vi "Set Navigation.vi"(9 "Enum":T1, 10 "Back":refnum<vi>, 11 "Next":refnum<vi>) -> ()   [LabVIEW 2021]
uses:
  Control/Navigation Control.ctl
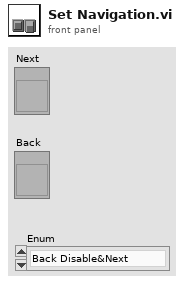
[diagram p1: front panel]
types:
  T1 = typedef "Navigation Control.ctl" = enum16{"Back Disable&Next", "Back Enable&Finish Disable", "Back Enable&Next", "Back Diable&Finish", "Back Enable&Finish", "Back Enable&Next Disable", "Back Disable&Next Disable"}
  T2 = enum8{"Enabled", "Disabled", "Disabled and Grayed Out"}
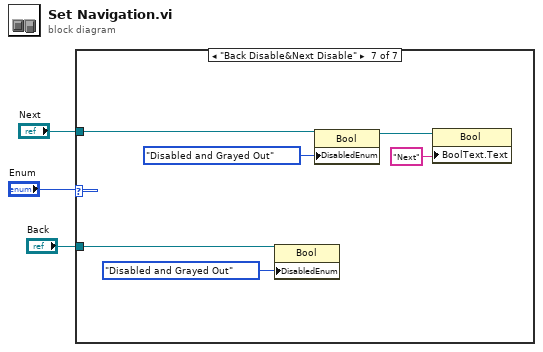
[diagram p0: block diagram]
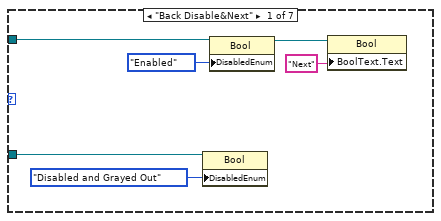
[diagram p2: hidden frame]
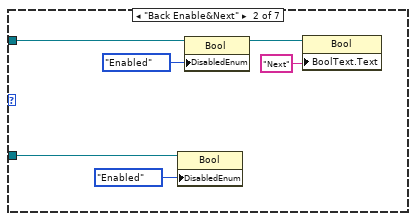
[diagram p3: hidden frame]
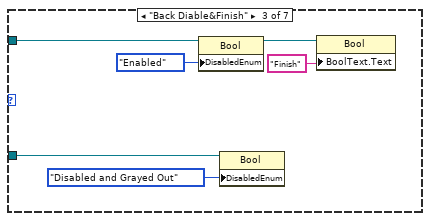
[diagram p4: hidden frame]
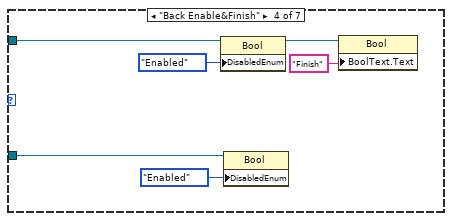
[diagram p5: hidden frame]
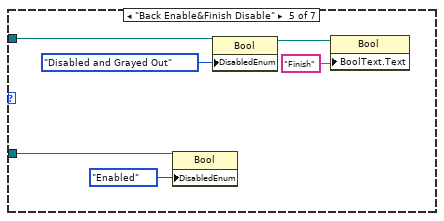
[diagram p6: hidden frame]
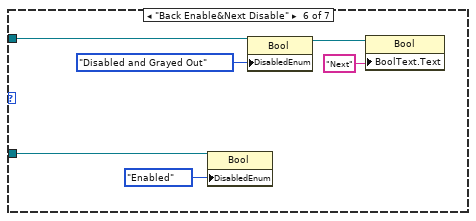
[diagram p7: hidden frame]
diagram:
  n1 = case shown="\"Back Disable&Next Disable\"" "Enum" {
    tunnel: "Back" -> [w4 w15 w16 w22 w28 w34 w40]
    tunnel: "Next" -> [w5 w14 w17 w23 w29 w35 w41]
    frame "Back Disable&Next" {
      n2 = property class="Bool"(reference=w4, "DisabledEnum"=T2."Disabled and Grayed Out" ("Disabled")) -> ()  [unwired: 1 in, 2 out]
      n3 = property class="Bool"(reference=w5, "DisabledEnum"=T2."Enabled" ("Disabled")) -> (reference out=w7:refnum<vi>)  [unwired: 1 in, 1 out]
      n4 = property class="Bool"(reference=w7, "BoolText.Text"="Next" ("Boolean Text.Text")) -> ()  [unwired: 1 in, 2 out]
    }
    frame "Back Enable&Next" {
      n5 = property class="Bool"(reference=w15, "DisabledEnum"=T2."Enabled" ("Disabled")) -> ()  [unwired: 1 in, 2 out]
      n6 = property class="Bool"(reference=w14, "DisabledEnum"=T2."Enabled" ("Disabled")) -> (reference out=w11:refnum<vi>)  [unwired: 1 in, 1 out]
      n7 = property class="Bool"(reference=w11, "BoolText.Text"="Next" ("Boolean Text.Text")) -> ()  [unwired: 1 in, 2 out]
    }
    frame "Back Diable&Finish" {
      n8 = property class="Bool"(reference=w17, "DisabledEnum"=T2."Enabled" ("Disabled")) -> (reference out=w19:refnum<vi>)  [unwired: 1 in, 1 out]
      n9 = property class="Bool"(reference=w16, "DisabledEnum"=T2."Disabled and Grayed Out" ("Disabled")) -> ()  [unwired: 1 in, 2 out]
      n10 = property class="Bool"(reference=w19, "BoolText.Text"="Finish" ("Boolean Text.Text")) -> ()  [unwired: 1 in, 2 out]
    }
    frame "Back Enable&Finish" {
      n11 = property class="Bool"(reference=w23, "DisabledEnum"=T2."Enabled" ("Disabled")) -> (reference out=w25:refnum<vi>)  [unwired: 1 in, 1 out]
      n12 = property class="Bool"(reference=w22, "DisabledEnum"=T2."Enabled" ("Disabled")) -> ()  [unwired: 1 in, 2 out]
      n13 = property class="Bool"(reference=w25, "BoolText.Text"="Finish" ("Boolean Text.Text")) -> ()  [unwired: 1 in, 2 out]
    }
    frame "Back Enable&Finish Disable" {
      n14 = property class="Bool"(reference=w28, "DisabledEnum"=T2."Enabled" ("Disabled")) -> ()  [unwired: 1 in, 2 out]
      n15 = property class="Bool"(reference=w29, "DisabledEnum"=T2."Disabled and Grayed Out" ("Disabled")) -> (reference out=w31:refnum<vi>)  [unwired: 1 in, 1 out]
      n16 = property class="Bool"(reference=w31, "BoolText.Text"="Finish" ("Boolean Text.Text")) -> ()  [unwired: 1 in, 2 out]
    }
    frame "Back Enable&Next Disable" {
      n17 = property class="Bool"(reference=w34, "DisabledEnum"=T2."Enabled" ("Disabled")) -> ()  [unwired: 1 in, 2 out]
      n18 = property class="Bool"(reference=w35, "DisabledEnum"=T2."Disabled and Grayed Out" ("Disabled")) -> (reference out=w37:refnum<vi>)  [unwired: 1 in, 1 out]
      n19 = property class="Bool"(reference=w37, "BoolText.Text"="Next" ("Boolean Text.Text")) -> ()  [unwired: 1 in, 2 out]
    }
    frame "Back Disable&Next Disable" {
      n20 = property class="Bool"(reference=w40, "DisabledEnum"=T2."Disabled and Grayed Out" ("Disabled")) -> ()  [unwired: 1 in, 2 out]
      n21 = property class="Bool"(reference=w41, "DisabledEnum"=T2."Disabled and Grayed Out" ("Disabled")) -> (reference out=w43:refnum<vi>)  [unwired: 1 in, 1 out]
      n22 = property class="Bool"(reference=w43, "BoolText.Text"="Next" ("Boolean Text.Text")) -> ()  [unwired: 1 in, 2 out]
    }
  }
